vi "Run cmd File.vi"() -> ()   [LabVIEW 2017]
panel:
  out "resulting string":string
  out "standard output":string
  out "Error out":errorcluster
  in  "Error in":errorcluster caption="Error in (no error)"
  in  "Path":path
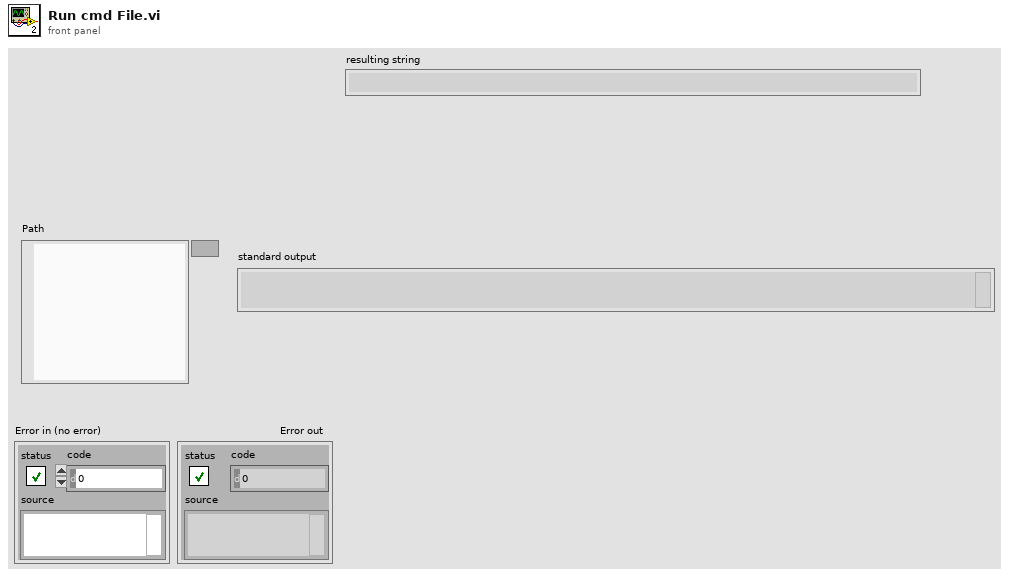
[diagram p1: front panel]
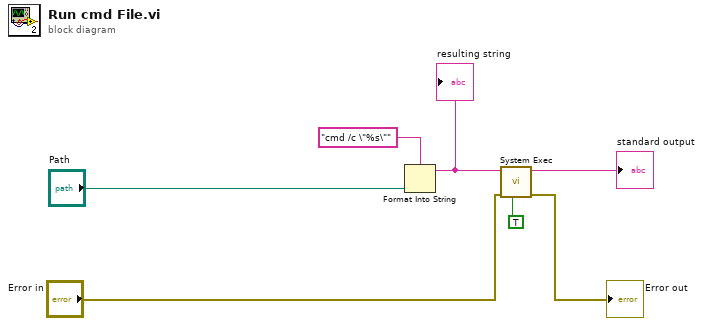
[diagram p0: block diagram]
diagram:
  n1 = Format Into String(format string="cmd /c \"%s\"", "Path") -> (resulting string=w2:string)  [unwired: 2 in, 1 out]
  "resulting string" <- w2
  n2 = call <vilib>:"System Exec.vi"("run minimized? (F)"=TRUE, "error in (no error)"="Error in", "command line"=w2) -> ("error out"=→"Error out":errorcluster, "standard output"=→"standard output":string)  [unwired: 5 in, 2 out]
